vi "Rename Object By ID.vi"(8 "error in (no error)":errorcluster, 9 "Name":string, 10 "ID":i32=-1, 11 "Objects in":refnum<class "Objects.lvclass">) -> (0 "error out":errorcluster, 3 "Objects out":refnum<class "Objects.lvclass">)   [LabVIEW 2019, in "HierDAL Library.lvlib" / "Database.lvlib" / "Repositories.lvlib" / "Objects.lvclass"]
uses:
  Objects.lvclass
  Objects.lvclass/Objects.ctl
  Database Manager Class/Database Manager.lvclass
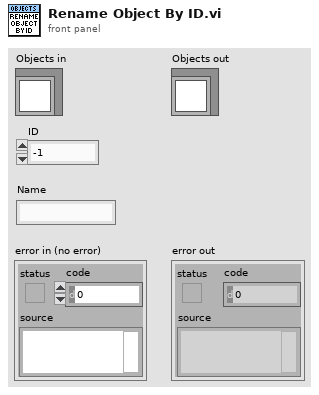
[diagram p1: front panel]
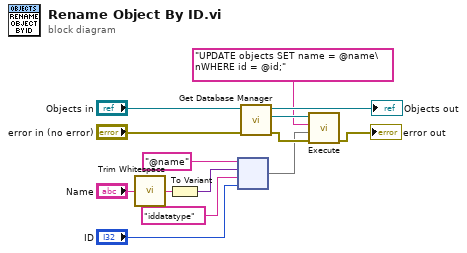
[diagram p0: block diagram]
diagram:
  n1 = call <vilib>:"Trim Whitespace.vi"("string"="Name") -> ("trimmed string"=w1:string)  [unwired: 1 in]
  n2 = To Variant(anything=w1) -> (Variant=w8:variant)
  n3 = node("@name" ("key"), w8, "iddatatype" ("key"), "ID") -> (w3:map{string, variant})
  n4 = call "Get Database Manager.vi"("error in (no error)"="error in (no error)", "Objects in"="Objects in") -> ("error out"=w11:errorcluster, "Database Manager"=w10:refnum<class "Database Manager.lvclass">, "Objects out"=→"Objects out":refnum<class "Objects.lvclass">)  [unwired: 7 in]
  n5 = call-dynamic "Execute.vi"("error in (no error)"=w11, "Parameters"=w3, "Query"="UPDATE objects SET name = @name\nWHERE id = @id;", "Database Manager in"=w10) -> ("error out"=→"error out":errorcluster)  [unwired: 6 in, 1 out]
